vi "GetSMUSense.vi"(7 "SMU":T1, 8 "Error In":errorcluster, 11 "Kiethley 2602 In":refnum<visa-resource-name>) -> (0 "Error Out":errorcluster, 2 "SMU Sense":T2, 3 "Keithley 2602 Out":refnum<visa-resource-name>)   [LabVIEW 2012, in "Keithley-2602.lvlib"]
uses:
  Keithley-2602.lvlib
  Controls/SMUSense.ctl
  Controls/SMU.ctl
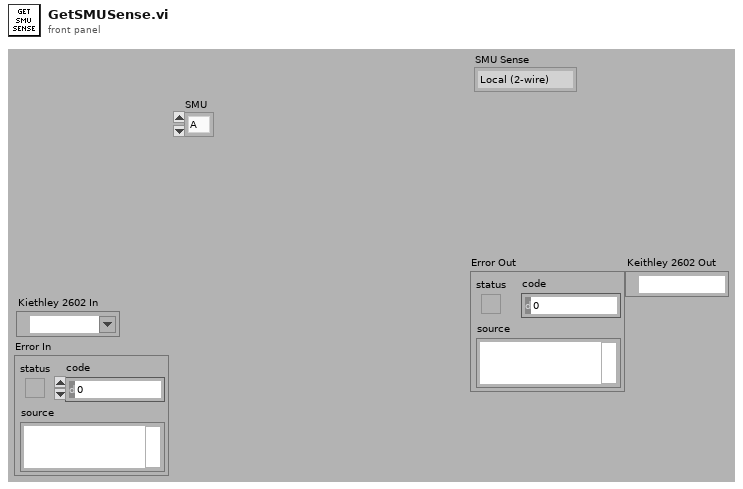
[diagram p1: front panel]
types:
  T1 = typedef "Keithley-2602.lvlib/SMU.ctl" = enum16{"A", "B"}
  T2 = typedef "Keithley-2602.lvlib/SMUSense.ctl" = enum16{"Local (2-wire)", "Remote (4-wire)", "Calibration"}
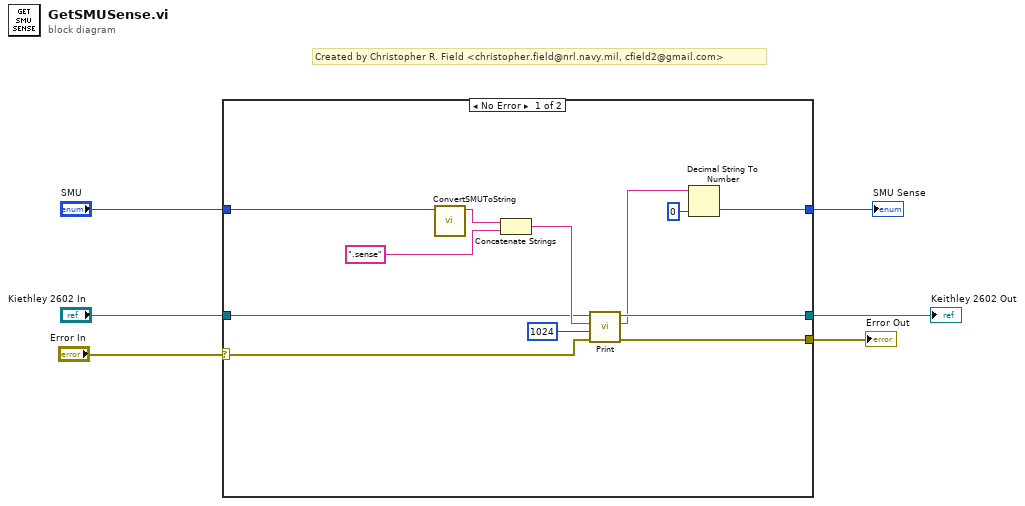
[diagram p0: block diagram]
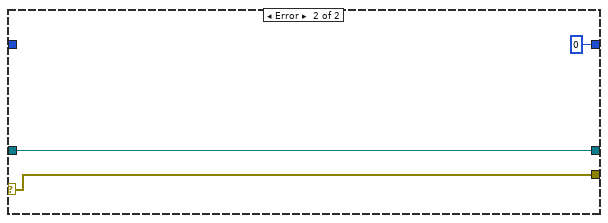
[diagram p2: hidden frame]
diagram:
  # "Created by Christopher R. Field <christopher.field@nrl.navy.mil, cfield2@gmail.com>"
  n1 = case shown="No Error" "Error In" {
    selector: "Error In" -> [w7 w20]
    tunnel: "Kiethley 2602 In" -> [w14 w21]
    tunnel: [w13 w20] -> w5
    tunnel: [w12 w21] -> w4
    tunnel: [w9 u16 0] -> w3
    tunnel: "SMU" -> [w8 _]
    frame No Error {
      n2 = call "ConvertSMUToString.vi"("SMU"=w8) -> ("Channel"=w18:string)  [unwired: 10 in]
      n3 = Concatenate Strings(w18, ".sense") -> (w16:string)
      n4 = call "Print.vi"("Error In"=w7, "Byte Count"=u32 1024, "Attribute"=w16, "Kiethley 2602 In"=w14) -> ("Error Out"=w13:errorcluster, "Output"=w11:string, "Keithley 2602 Out"=w12:refnum<visa-resource-name>)  [unwired: 5 in]
      n5 = Decimal String To Number(string=w11, default (0L)=u16 0 ("default (0 I32)")) -> (number=w9:u16)  [unwired: 1 in, 1 out]
    }
    frame Error {
    }
  }
  "Error Out" <- w5
  "Keithley 2602 Out" <- w4
  "SMU Sense" <- w3
